vi "W4q1.vi"() -> ()   [LabVIEW 2021]
panel:
  in  "Enum":T1(ring)
  out "Waveform Graph":dynamicdata(graph)
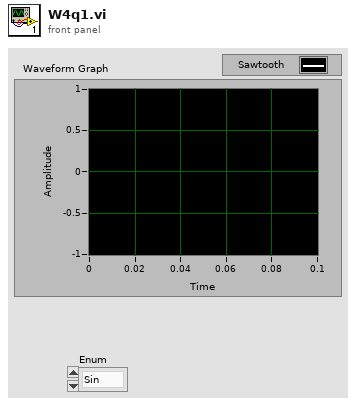
[diagram p1: front panel]
types:
  T1 = enum16{"Sin", "Triangular", "square", "Sawtooth", "DC"}
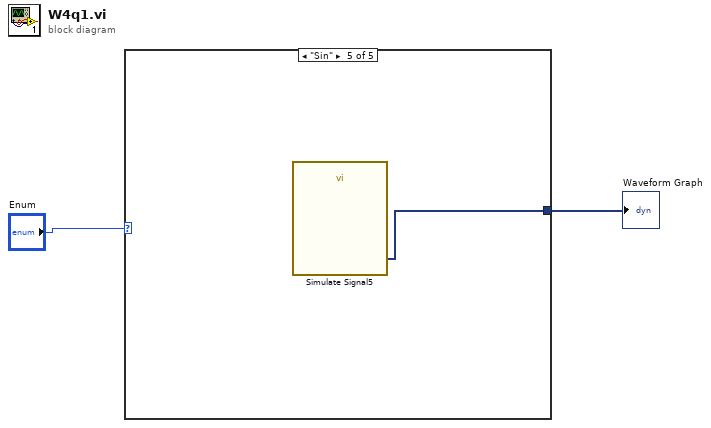
[diagram p0: block diagram]
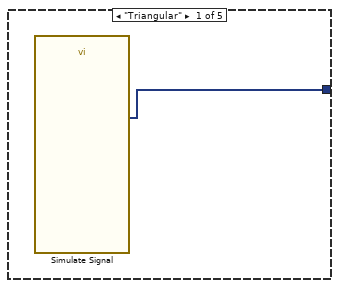
[diagram p2: hidden frame]
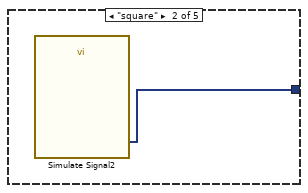
[diagram p3: hidden frame]
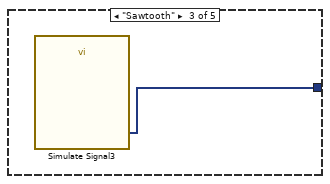
[diagram p4: hidden frame]
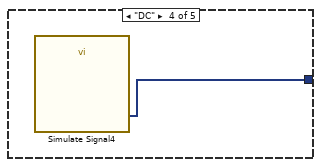
[diagram p5: hidden frame]
diagram:
  n1 = case shown="\"Sin\"" "Enum" {
    tunnel: [w3 w4 w5 w6 w7] -> w1
    frame "Triangular" {
      n2 = call "Simulate Signal"() -> ("Triangle"=w3:dynamicdata)  [unwired: 14 in, 1 out]
    }
    frame "square" {
      n3 = call "Simulate Signal2"() -> ("Square"=w4:dynamicdata)  [unwired: 14 in, 1 out]
    }
    frame "Sawtooth" {
      n4 = call "Simulate Signal3"() -> ("Sawtooth"=w5:dynamicdata)  [unwired: 14 in, 1 out]
    }
    frame "DC" {
      n5 = call "Simulate Signal4"() -> ("DC"=w6:dynamicdata)  [unwired: 14 in, 1 out]
    }
    frame "Sin" {
      n6 = call "Simulate Signal5"() -> ("Sine"=w7:dynamicdata)  [unwired: 14 in, 1 out]
    }
  }
  "Waveform Graph" <- w1
